vi "VI Tree.vi"   [LabVIEW 2021, in "Field_RnD_Services_LIBSSH2_Toolkit.lvlib"]
doc: "Shows all of the public VIs for the toolkit grouped by LabVIEW class in the block diagram."
uses:
  220524-VNA RP FLAT.llb/Field_RnD_Services_LIBSSH2_Toolkit.lvlib
  220524-VNA RP FLAT.llb/SSH.lvclass
  220524-VNA RP FLAT.llb/Agent Identity.lvclass
  220524-VNA RP FLAT.llb/Agent.lvclass
  220524-VNA RP FLAT.llb/Channel.lvclass
  220524-VNA RP FLAT.llb/File Info.lvclass
  220524-VNA RP FLAT.llb/Known Host.lvclass
  220524-VNA RP FLAT.llb/Destroy to Listener.vi
  Field_RnD_Services_LIBSSH2_Toolkit.lvlib_File Info/Create from Session.vi
  220524-VNA RP FLAT.llb/Create from Listener.vi
  220524-VNA RP FLAT.llb/Create from Agent.vi
  Field_RnD_Services_LIBSSH2_Toolkit.lvlib_Agent/Create from Session.vi
  Field_RnD_Services_LIBSSH2_Toolkit.lvlib_Agent/Destroy to Session.vi
  220524-VNA RP FLAT.llb/Destroy to Agent.vi
  220524-VNA RP FLAT.llb/Known Hosts.lvclass
  220524-VNA RP FLAT.llb/Listener.lvclass
  220524-VNA RP FLAT.llb/Session.lvclass
  220524-VNA RP FLAT.llb/SFTP Attributes.lvclass
  220524-VNA RP FLAT.llb/SFTP Directory.lvclass
  220524-VNA RP FLAT.llb/SFTP File.lvclass
  220524-VNA RP FLAT.llb/SFTP.lvclass
  Field_RnD_Services_LIBSSH2_Toolkit.lvlib_Session/Create from SSH.vi
  220524-VNA RP FLAT.llb/Password Authentication.vi
  Field_RnD_Services_LIBSSH2_Toolkit.lvlib_Session/Destroy to SSH.vi
  Field_RnD_Services_LIBSSH2_Toolkit.lvlib_Known Hosts/Create from Session.vi
  220524-VNA RP FLAT.llb/Destroy to Known Hosts.vi
  220524-VNA RP FLAT.llb/Create from Known Hosts.vi
  Field_RnD_Services_LIBSSH2_Toolkit.lvlib_Known Hosts/Destroy to Session.vi
  Field_RnD_Services_LIBSSH2_Toolkit.lvlib_Listener/Destroy to Session.vi
  Field_RnD_Services_LIBSSH2_Toolkit.lvlib_Listener/Create from Session.vi
  Field_RnD_Services_LIBSSH2_Toolkit.lvlib_SFTP File/Close to SFTP.vi
  Field_RnD_Services_LIBSSH2_Toolkit.lvlib_SFTP Directory/Open from SFTP.vi
  Field_RnD_Services_LIBSSH2_Toolkit.lvlib_SFTP File/Open from SFTP.vi
  Field_RnD_Services_LIBSSH2_Toolkit.lvlib_SFTP/Create from Session.vi
  Field_RnD_Services_LIBSSH2_Toolkit.lvlib_SFTP/Destroy to Session.vi
  220524-VNA RP FLAT.llb/Resolve Symbolic Link.vi
  Field_RnD_Services_LIBSSH2_Toolkit.lvlib_SFTP Directory/Close to SFTP.vi
  220524-VNA RP FLAT.llb/Destroy to SFTP Directory.vi
  220524-VNA RP FLAT.llb/Create from SFTP Directory.vi
  Field_RnD_Services_LIBSSH2_Toolkit.lvlib_File Info/Destroy to Session.vi
panel:
  # "Copyright (c) 2019 Field R&D Services, LLC\n\nLicensed under the Apache License, Version 2.0 (the \"License\"); you may not use this file except in compliance with the License.  You may obtain a copy of the License at\n\nhttp://www.apache.org/licenses/LICENSE-2.0\n\nUnless required by applicable law or agreed to in writing, software distributed under the License is distributed on an \"AS IS\" BASIS, WITHOUT WARRANTIES OR CONDITIONS OF ANY KIND, either express or implied.  See the License for the specific language governing permissions and limitations under the License.\n\nLIBSSH2-LabVIEW is licensed under either the BSD-3-Clause (https://opensource.org/licenses/BSD-3-Clause) or the Apache-2.0 license, http://www.apache.org/licenses/LICENSE-2.0, and it contains statically compiled code from the libssh2 (https://github.com/libssh2/libssh2) and OpenSSL (https://github.com/openssl/openssl) projects, which are licensed under the MIT license (https://github.com/libssh2/libssh2/blob/master/COPYING) and the Apache-2.0 license, https://github.com/openssl/openssl/blob/master/LICENSE, respectively."
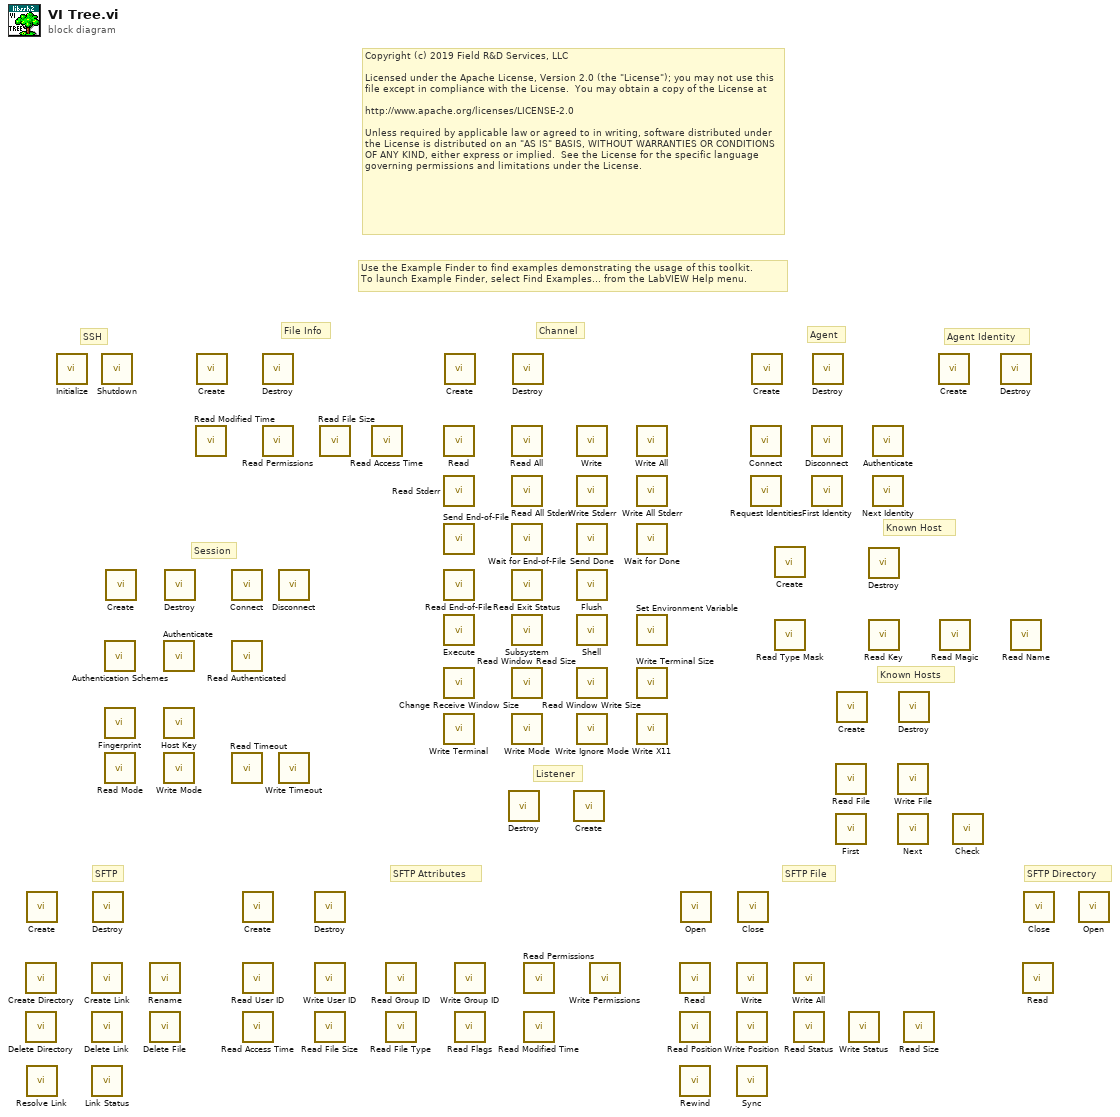
[diagram p0: block diagram]
diagram:
  # "SFTP"
  # "SFTP File"
  # "SFTP Directory"
  # "SFTP Attributes"
  # "Use the Example Finder to find examples demonstrating the usage of this toolkit.\nTo launch Example Finder, select Find Examples... from the LabVIEW Help menu."
  # "Session"
  # "Listener"
  # "Known Hosts"
  # "Known Host"
  # "File Info"
  # "Channel"
  # "Agent"
  # "Agent Identity"
  # "SSH"
  # "Copyright (c) 2019 Field R&D Services, LLC\n\nLicensed under the Apache License, Version 2.0 (the \"License\"); you may not use this file except in compliance with the License.  You may obtain a copy of the License at\n\nhttp://www.apache.org/licenses/LICENSE-2.0\n\nUnless required by applicable law or agreed to in writing, software distributed under the License is distributed on an \"AS IS\" BASIS, WITHOUT WARRANTIES OR CONDITIONS OF ANY KIND, either express or implied.  See the License for the specific language governing permissions and limitations under the License."
  n1 = call "Create Directory.vi"() -> ()  [unwired: 10 in, 2 out]
  n2 = call "Delete Directory.vi"() -> ()  [unwired: 10 in, 2 out]
  n3 = call-poly "Create.vi"() -> ()  [unwired: 10 in, 2 out]
  n4 = call-poly "Resolve Link.vi"() -> ()  [unwired: 9 in, 3 out]
  n5 = call "Initialize.vi"() -> ()  [unwired: 10 in, 2 out]
  n6 = call "Create Link.vi"() -> ()  [unwired: 10 in, 2 out]
  n7 = call "Delete Link.vi"() -> ()  [unwired: 10 in, 2 out]
  n8 = call "Link Status.vi"() -> ()  [unwired: 9 in, 3 out]
  n9 = call-poly "Destroy.vi"() -> ()  [unwired: 10 in, 2 out]
  n10 = call "Shutdown.vi"() -> ()  [unwired: 11 in, 1 out]
  n11 = call "Authentication Schemes.vi"() -> ()  [unwired: 9 in, 3 out]
  n12 = call "Fingerprint.vi"() -> ()  [unwired: 9 in, 3 out]
  n13 = call "Read Mode.vi"() -> ()  [unwired: 9 in, 3 out]
  n14 = call-poly "Create.vi"() -> ()  [unwired: 10 in, 2 out]
  n15 = call "Rename.vi"() -> ()  [unwired: 10 in, 2 out]
  n16 = call "Delete File.vi"() -> ()  [unwired: 10 in, 2 out]
  n17 = call-poly "Authenticate.vi"() -> ()  [unwired: 10 in, 2 out]
  n18 = call "Host Key.vi"() -> ()  [unwired: 8 in, 4 out]
  n19 = call "Write Mode.vi"() -> ()  [unwired: 10 in, 2 out]
  n20 = call-poly "Destroy.vi"() -> ()  [unwired: 10 in, 2 out]
  n21 = call "Read Modified Time.vi"() -> ()  [unwired: 9 in, 3 out]
  n22 = call-poly "Create.vi"() -> ()  [unwired: 9 in, 3 out]
  n23 = call "Connect.vi"() -> ()  [unwired: 10 in, 2 out]
  n24 = call "Read Authenticated.vi"() -> ()  [unwired: 9 in, 3 out]
  n25 = call "Read Timeout.vi"() -> ()  [unwired: 9 in, 3 out]
  n26 = call-poly "Create.vi"() -> ()  [unwired: 9 in, 3 out]
  n27 = call "Read User ID.vi"() -> ()  [unwired: 9 in, 3 out]
  n28 = call "Read Access Time.vi"() -> ()  [unwired: 9 in, 3 out]
  n29 = call-poly "Destroy.vi"() -> ()  [unwired: 10 in, 2 out]
  n30 = call "Read Permissions.vi"() -> ()  [unwired: 9 in, 3 out]
  n31 = call "Disconnect.vi"() -> ()  [unwired: 10 in, 2 out]
  n32 = call "Write Timeout.vi"() -> ()  [unwired: 10 in, 2 out]
  n33 = call-poly "Destroy.vi"() -> ()  [unwired: 10 in, 2 out]
  n34 = call "Write User ID.vi"() -> ()  [unwired: 10 in, 2 out]
  n35 = call "Read File Size.vi"() -> ()  [unwired: 9 in, 3 out]
  n36 = call "Read File Size.vi"() -> ()  [unwired: 9 in, 3 out]
  n37 = call "Read Access Time.vi"() -> ()  [unwired: 9 in, 3 out]
  n38 = call "Read Group ID.vi"() -> ()  [unwired: 9 in, 3 out]
  n39 = call "Read File Type.vi"() -> ()  [unwired: 9 in, 3 out]
  n40 = call "Read.vi"() -> ()  [unwired: 9 in, 3 out]
  n41 = call "Read Stderr.vi"() -> ()  [unwired: 9 in, 3 out]
  n42 = call "Send End-of-File.vi"() -> ()  [unwired: 10 in, 2 out]
  n43 = call "Read End-of-File.vi"() -> ()  [unwired: 9 in, 3 out]
  n44 = call "Execute.vi"() -> ()  [unwired: 10 in, 2 out]
  n45 = call "Change Receive Window Size.vi"() -> ()  [unwired: 9 in, 3 out]
  n46 = call "Write Terminal.vi"() -> ()  [unwired: 10 in, 2 out]
  n47 = call-poly "Create.vi"() -> ()  [unwired: 10 in, 2 out]
  n48 = call "Write Group ID.vi"() -> ()  [unwired: 10 in, 2 out]
  n49 = call "Read Flags.vi"() -> ()  [unwired: 9 in, 3 out]
  n50 = call-poly "Destroy.vi"() -> ()  [unwired: 10 in, 2 out]
  n51 = call "Read All.vi"() -> ()  [unwired: 8 in, 4 out]
  n52 = call "Read All Stderr.vi"() -> ()  [unwired: 8 in, 4 out]
  n53 = call "Wait for End-of-File.vi"() -> ()  [unwired: 10 in, 2 out]
  n54 = call "Read Exit Status.vi"() -> ()  [unwired: 9 in, 3 out]
  n55 = call "Subsystem.vi"() -> ()  [unwired: 10 in, 2 out]
  n56 = call "Read Window Read Size.vi"() -> ()  [unwired: 9 in, 3 out]
  n57 = call "Write Mode.vi"() -> ()  [unwired: 10 in, 2 out]
  n58 = call-poly "Destroy.vi"() -> ()  [unwired: 10 in, 2 out]
  n59 = call "Read Permissions.vi"() -> ()  [unwired: 9 in, 3 out]
  n60 = call "Read Modified Time.vi"() -> ()  [unwired: 9 in, 3 out]
  n61 = call-poly "Create.vi"() -> ()  [unwired: 10 in, 2 out]
  n62 = call "Write.vi"() -> ()  [unwired: 9 in, 3 out]
  n63 = call "Write Stderr.vi"() -> ()  [unwired: 9 in, 3 out]
  n64 = call "Send Done.vi"() -> ()  [unwired: 10 in, 2 out]
  n65 = call "Flush.vi"() -> ()  [unwired: 10 in, 2 out]
  n66 = call "Shell.vi"() -> ()  [unwired: 10 in, 2 out]
  n67 = call "Read Window Write Size.vi"() -> ()  [unwired: 9 in, 3 out]
  n68 = call "Write Ignore Mode.vi"() -> ()  [unwired: 10 in, 2 out]
  n69 = call "Write Permissions.vi"() -> ()  [unwired: 10 in, 2 out]
  n70 = call "Write All.vi"() -> ()  [unwired: 8 in, 4 out]
  n71 = call "Write All Stderr.vi"() -> ()  [unwired: 8 in, 4 out]
  n72 = call "Wait for Done.vi"() -> ()  [unwired: 10 in, 2 out]
  n73 = call "Set Environment Variable.vi"() -> ()  [unwired: 10 in, 2 out]
  n74 = call "Write Terminal Size.vi"() -> ()  [unwired: 10 in, 2 out]
  n75 = call "Write X11.vi"() -> ()  [unwired: 10 in, 2 out]
  n76 = call "Read.vi"() -> ()  [unwired: 9 in, 3 out]
  n77 = call "Read Position.vi"() -> ()  [unwired: 9 in, 3 out]
  n78 = call "Rewind.vi"() -> ()  [unwired: 10 in, 2 out]
  n79 = call-poly "Open.vi"() -> ()  [unwired: 10 in, 2 out]
  n80 = call "Write.vi"() -> ()  [unwired: 9 in, 3 out]
  n81 = call "Write Position.vi"() -> ()  [unwired: 10 in, 2 out]
  n82 = call "Sync.vi"() -> ()  [unwired: 10 in, 2 out]
  n83 = call-poly "Close.vi"() -> ()  [unwired: 9 in, 3 out]
  n84 = call "Connect.vi"() -> ()  [unwired: 10 in, 2 out]
  n85 = call "Request Identities.vi"() -> ()  [unwired: 10 in, 2 out]
  n86 = call-poly "Create.vi"() -> ()  [unwired: 10 in, 2 out]
  n87 = call-poly "Create.vi"() -> ()  [unwired: 9 in, 3 out]
  n88 = call "Read Type Mask.vi"() -> ()  [unwired: 9 in, 3 out]
  n89 = call "Write All.vi"() -> ()  [unwired: 9 in, 3 out]
  n90 = call "Read Status.vi"() -> ()  [unwired: 9 in, 3 out]
  n91 = call "Disconnect.vi"() -> ()  [unwired: 10 in, 2 out]
  n92 = call "First Identity.vi"() -> ()  [unwired: 8 in, 4 out]
  n93 = call-poly "Destroy.vi"() -> ()  [unwired: 10 in, 2 out]
  n94 = call "Read File.vi"() -> ()  [unwired: 9 in, 3 out]
  n95 = call "First.vi"() -> ()  [unwired: 8 in, 4 out]
  n96 = call-poly "Create.vi"() -> ()  [unwired: 10 in, 2 out]
  n97 = call "Write Status.vi"() -> ()  [unwired: 9 in, 3 out]
  n98 = call-poly "Destroy.vi"() -> ()  [unwired: 10 in, 2 out]
  n99 = call "Read Key.vi"() -> ()  [unwired: 9 in, 3 out]
  n100 = call "Authenticate.vi"() -> ()  [unwired: 9 in, 3 out]
  n101 = call "Next Identity.vi"() -> ()  [unwired: 7 in, 5 out]
  n102 = call "Write File.vi"() -> ()  [unwired: 10 in, 2 out]
  n103 = call "Next.vi"() -> ()  [unwired: 7 in, 5 out]
  n104 = call-poly "Destroy.vi"() -> ()  [unwired: 10 in, 2 out]
  n105 = call "Read Size.vi"() -> ()  [unwired: 9 in, 3 out]
  n106 = call-poly "Create.vi"() -> ()  [unwired: 9 in, 3 out]
  n107 = call "Read Magic.vi"() -> ()  [unwired: 9 in, 3 out]
  n108 = call "Check.vi"() -> ()  [unwired: 9 in, 3 out]
  n109 = call-poly "Destroy.vi"() -> ()  [unwired: 10 in, 2 out]
  n110 = call "Read Name.vi"() -> ()  [unwired: 9 in, 3 out]
  n111 = call "Read.vi"() -> ()  [unwired: 7 in, 5 out]
  n112 = call-poly "Close.vi"() -> ()  [unwired: 9 in, 3 out]
  n113 = call-poly "Open.vi"() -> ()  [unwired: 10 in, 2 out]
